vi "Verify Borders.vi"(7 "Column Number":i32, 8 "error in (no error)":errorcluster, 9 "Borders IN":T6={"Title Row Border"={"Line"={"Thickness"=0.5, "Color"=0}, "Column Borders [ ]"=[]}, "Datas Row Borders [ ]"=[]}, 11 "Predefined Borders":T1={"Borders"=0, "Title"={"Thickness"=1.0, "Line"=0, "Background "=16777226}, "Datas"={"Thickness"=0.5, "Line"=0, "Background "=16777215}}) -> (0 "error out":errorcluster, 2 "Borders OUT":T6={"Title Row Border"={"Line"={"Thickness"=0.5, "Color"=0}, "Column Borders [ ]"=[]}, "Datas Row Borders [ ]"=[{"Row"={"#"=0, "to #"=-1}, "Line"={"Thickness"=0.5, "Color"=0}, "Column Borders [ ]"=[]}]}, 4 "ms":u32)   [LabVIEW 2012]
doc: "Version 1.0\nDeveloped by Jean-Marc Simard\nCopyright © 2010, Exaprom Inc.\nAll rights reserved.\nLicense: BSD"
uses:
  Controls/Row Border Title.ctl
  Controls/Cell Border.ctl
  Controls/Row Borders [ ] Datas.ctl
  Controls/Row Predefined borders cluster.ctl
  Controls/Row Predefined borders.ctl
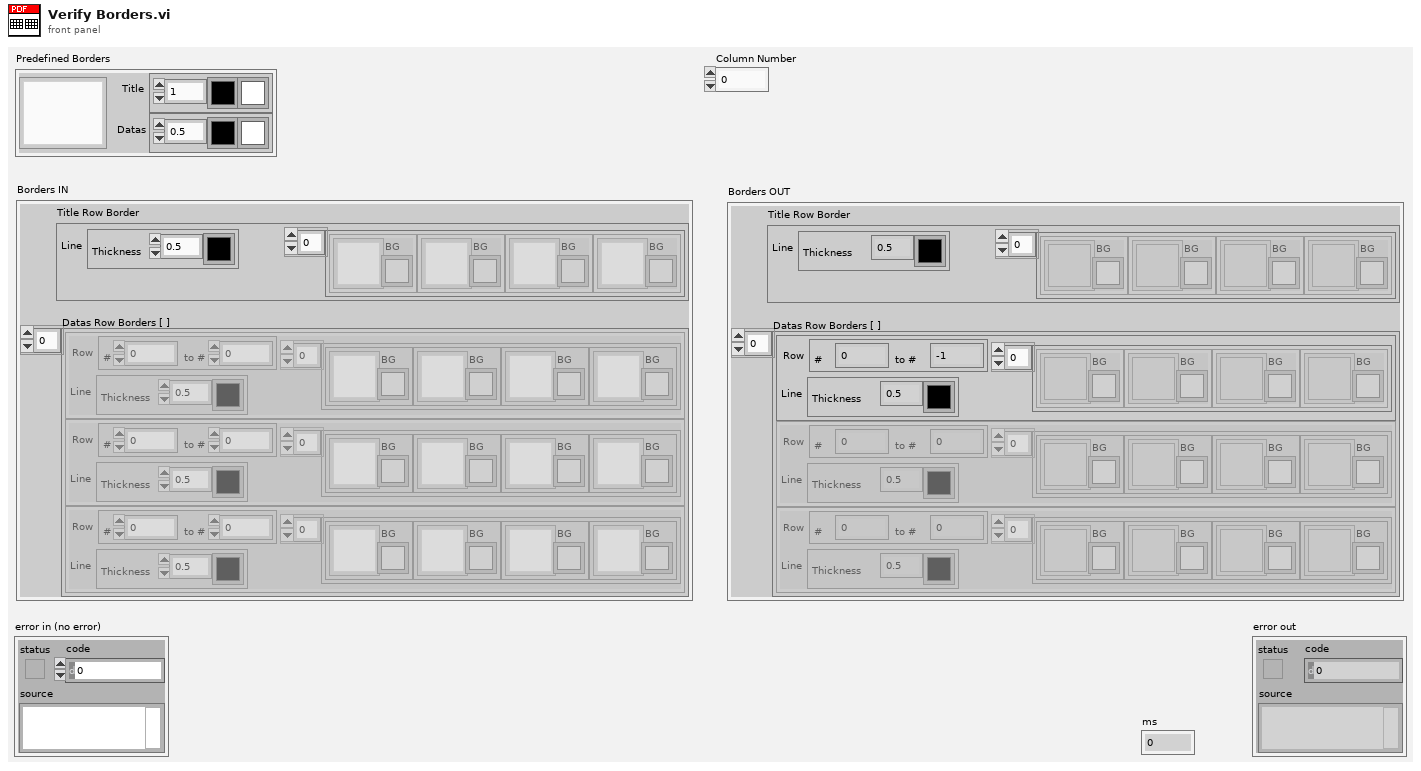
[diagram p1: front panel]
types:
  T1 = typedef "Row Predefined borders cluster.ctl" = cluster{"Borders":T2, "Title":cluster{"Thickness":sgl, "Line":u32, "Background ":u32}, "Datas":cluster{"Thickness":sgl, "Line":u32, "Background ":u32}}
  T2 = typedef "Row Predefined borders.ctl" = u16
  T3 = typedef "Row Border Title.ctl" = cluster{"Line":cluster{"Thickness":sgl, "Color":u32}, "Column Borders [ ]":cluster{"Cell Border":T4, "BG":u32}[]}
  T4 = typedef "Cell Border.ctl" = u16
  T5 = typedef "Row Borders [ ] Datas.ctl" = cluster{"Row":cluster{"#":i16, "to #":i16}, "Line":cluster{"Thickness":sgl, "Color":u32}, "Column Borders [ ]":cluster{"Cell Border":T4, "BG":u32}[]}[]
  T6 = cluster{"Title Row Border":T3, "Datas Row Borders [ ]":T5}
  T7 = cluster{"Row":cluster{"#":i16, "to #":i32}, "Line":cluster{"Thickness":sgl, "Color":u32}, "Column Borders [ ]":cluster{"Cell Border":T4, "BG":u32}[]}
  T8 = cluster{"Row":cluster{"#":i32, "to #":i32}, "Line":cluster{"Thickness":sgl, "Color":u32}, "Column Borders [ ]":cluster{"Cell Border":T4, "BG":u32}[]}
  T9 = cluster{"Row":cluster{"#":i16, "to #":i32}, "Line":cluster{"Thickness":sgl, "Color":u32}, "Column Borders [ ]":cluster{"Cell Border":T4, "BG":u32}[]}[]
  T10 = cluster{"Title Row Border":T3, cluster{"Row":cluster{"#":i16, "to #":i32}, "Line":cluster{"Thickness":sgl, "Color":u32}, "Column Borders [ ]":cluster{"Cell Border":T4, "BG":u32}[]}[]}
  T11 = cluster{"Row":cluster{"#":i32, "to #":i32}, "Line":cluster{"Thickness":sgl, "Color":u32}, "Column Borders [ ]":cluster{"Cell Border":T4, "BG":u32}[]}[]
  T12 = cluster{"Title Row Border":T3, cluster{"Row":cluster{"#":i32, "to #":i32}, "Line":cluster{"Thickness":sgl, "Color":u32}, "Column Borders [ ]":cluster{"Cell Border":T4, "BG":u32}[]}[]}
  T13 = cluster{"Row":cluster{"#":i16, "to #":i16}, "Line":cluster{"Thickness":sgl, "Color":u32}, "Column Borders [ ]":cluster{"Cell Border":T4, "BG":u32}[]}
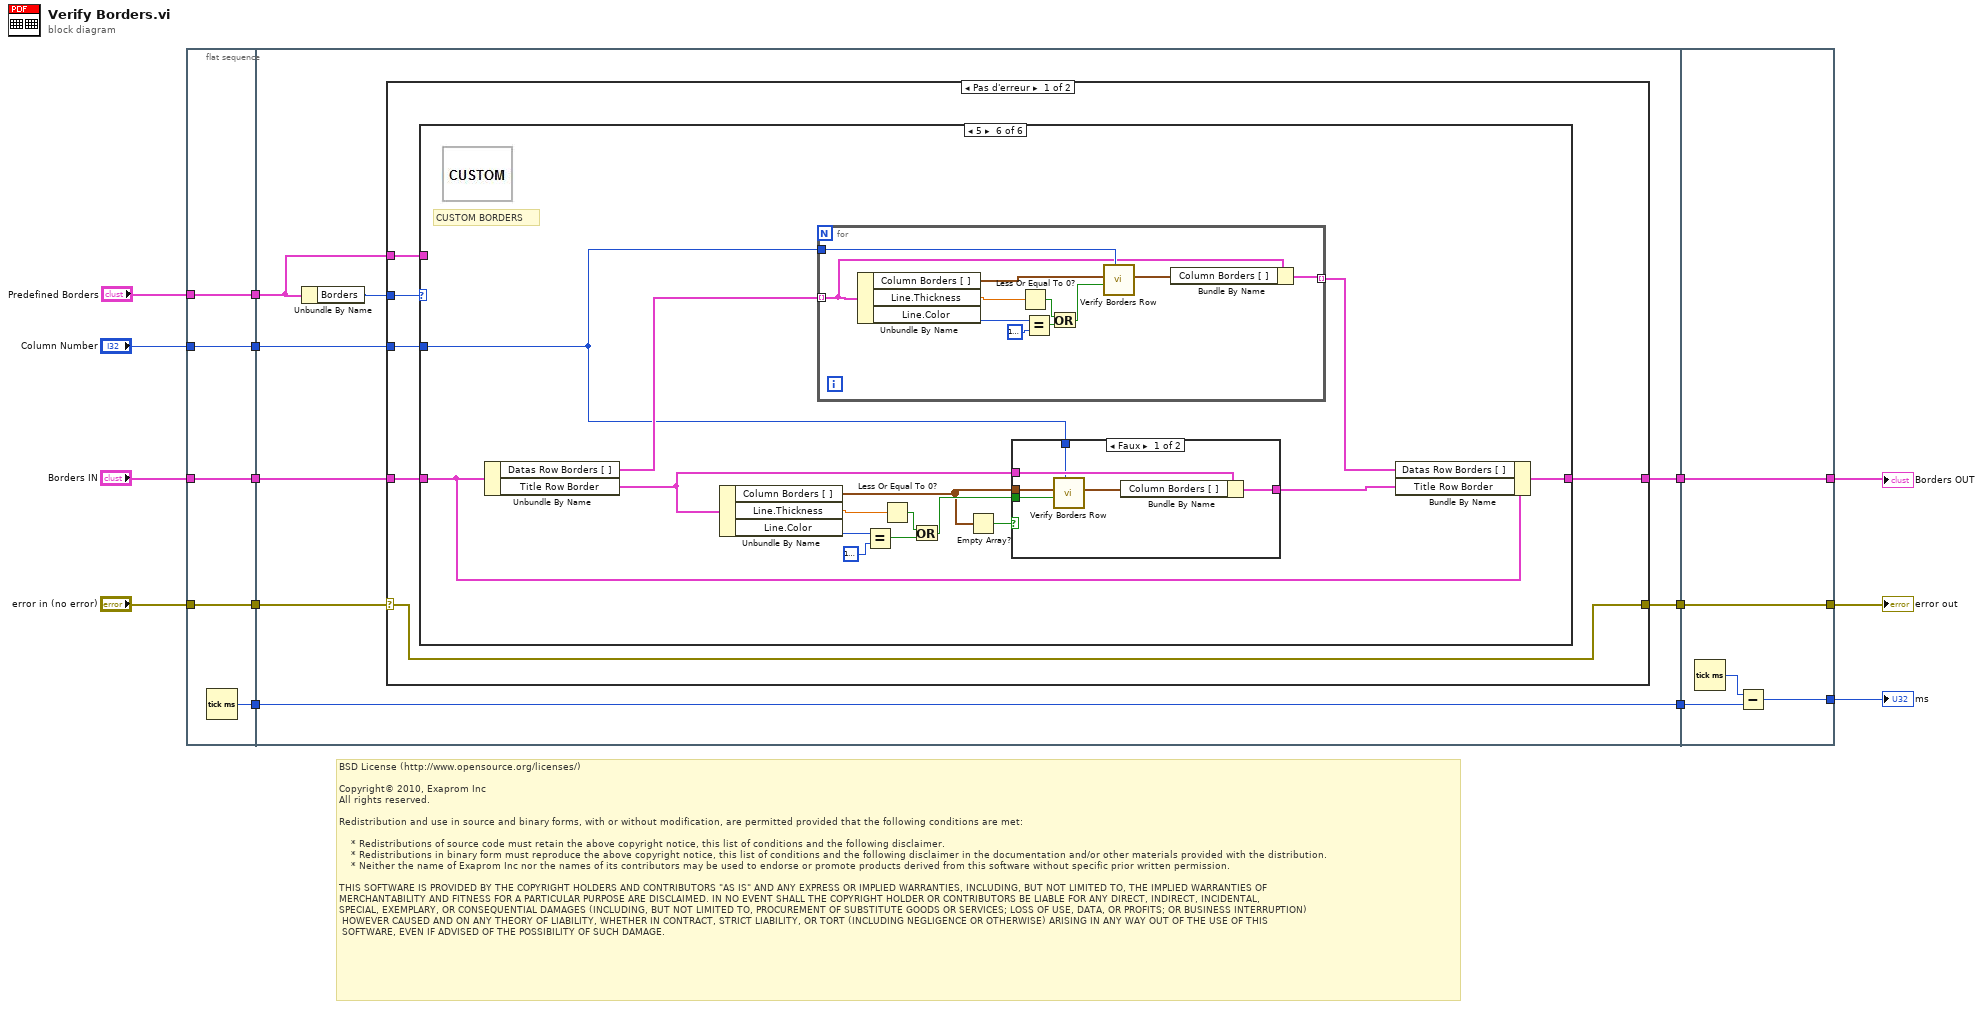
[diagram p0: block diagram]
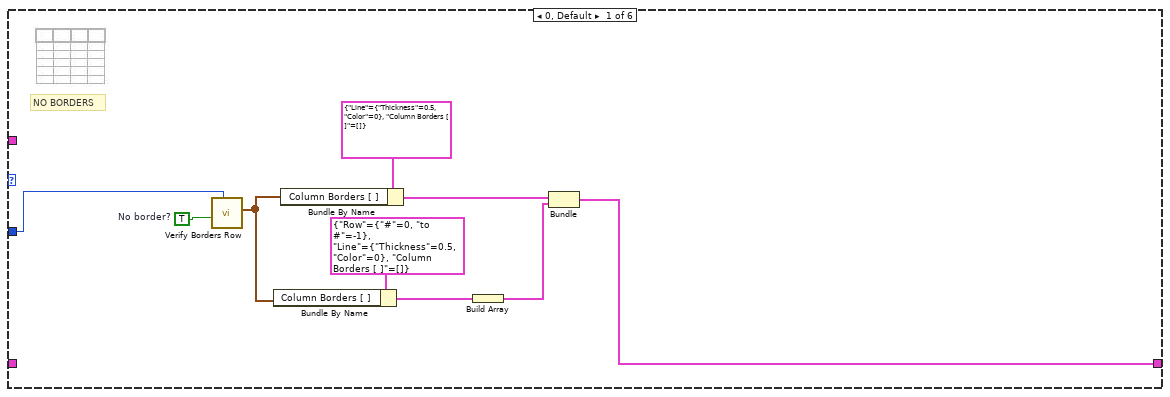
[diagram p2: hidden frame]
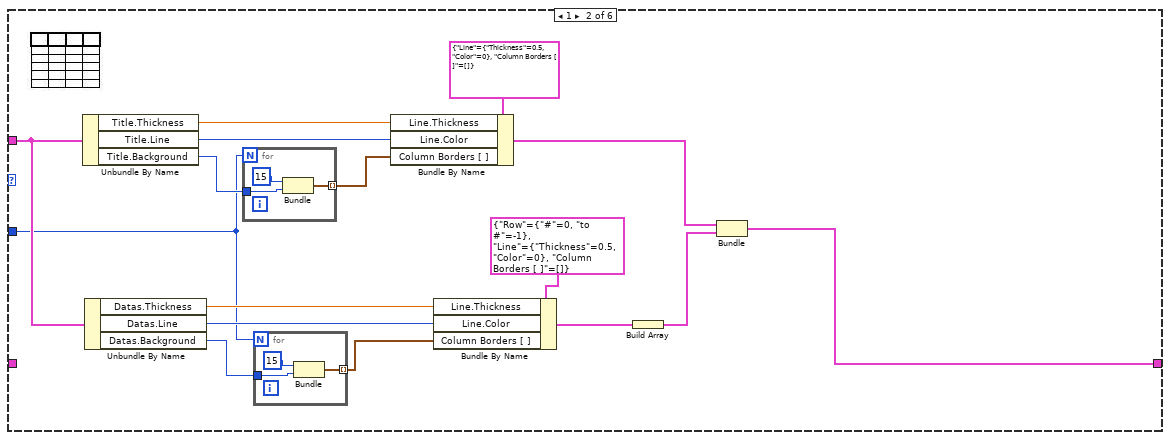
[diagram p3: hidden frame]
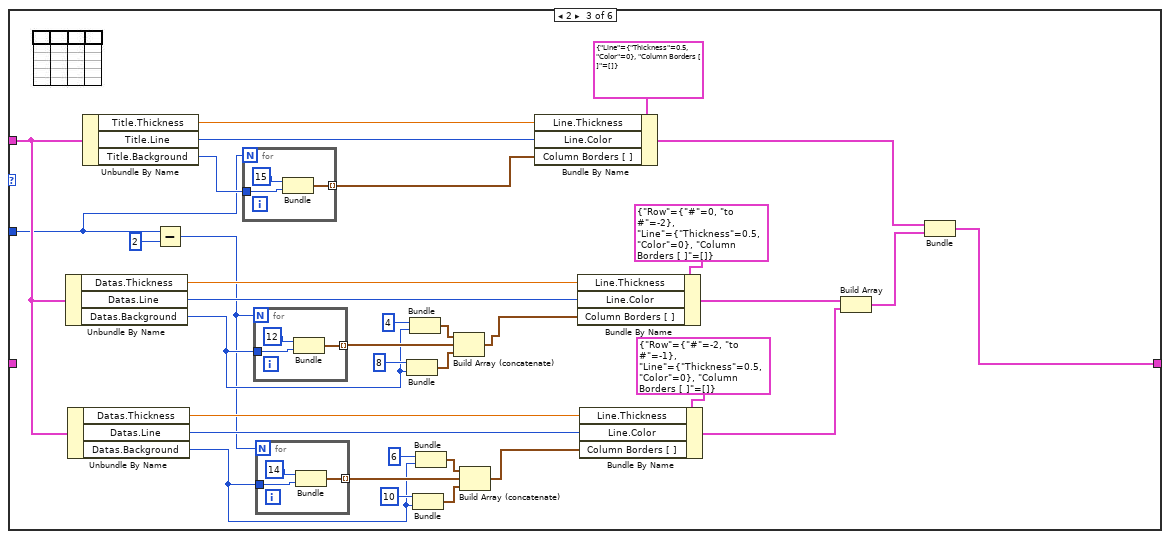
[diagram p4: hidden frame]
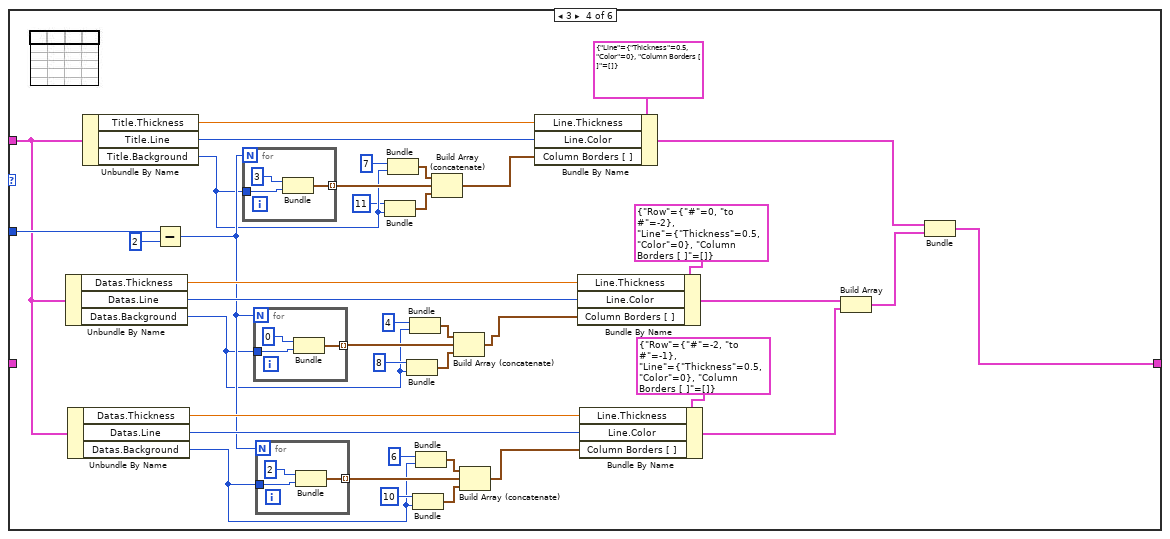
[diagram p5: hidden frame]
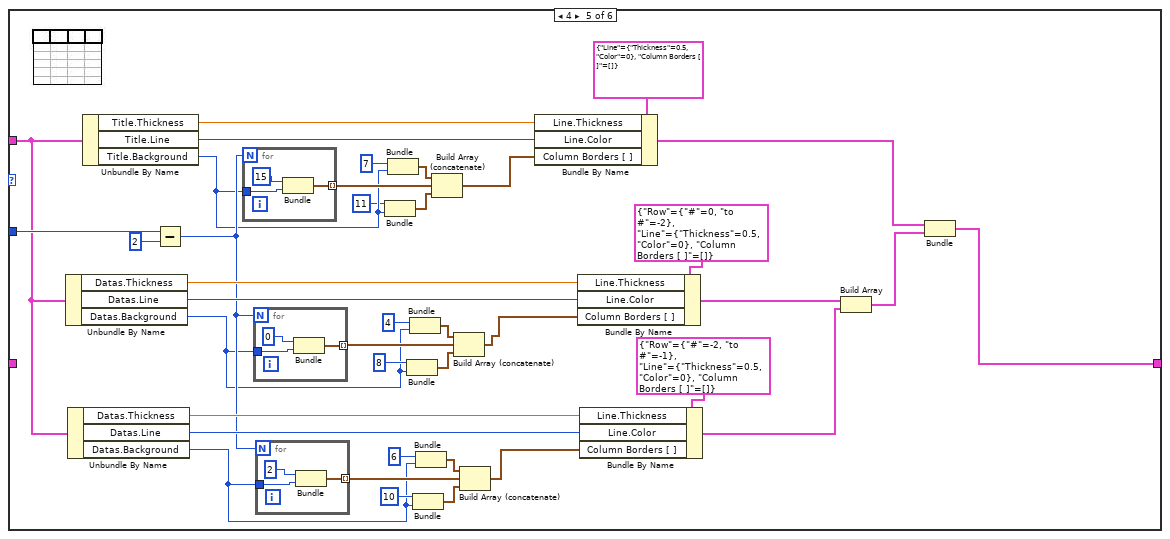
[diagram p6: hidden frame]
diagram:
  # "BSD License (http://www.opensource.org/licenses/)\n\nCopyright© 2010, Exaprom Inc\nAll rights reserved.\n\nRedistribution and use in source and binary forms, with or without modification, are permitted provided that the following conditions are met:\n\n    * Redistributions of source code must retain the above copyright notice, this list of conditions and the following disclaimer.\n    * Redistributions in binary form must reproduce the above copyright notice, this list of conditions and the following disclaimer in the documentation and/or other materials provided with the distribution.\n    * Neither the name of Exaprom Inc nor the names of its contributors may be used to endorse or promote products derived from this software without specific prior written permission.\n\nTHIS SOFTWARE IS PROVIDED BY THE COPYRIGHT HOLDERS AND CONTRIBUTORS \"AS IS\" AND ANY EXPRESS OR IMPLIED WARRANTIES, INCLUDING, BUT NOT LIMITED TO, THE IMPLIED WARRANTIES OF \nMERCHANTABILITY AND FITNESS FOR A PARTICULAR PURPOSE ARE DISCLAIMED. IN NO EVENT SHALL THE COPYRIGHT HOLDER OR CONTRIBUTORS BE LIABLE FOR ANY DIRECT, INDIRECT, INCIDENTAL,\nSPECIAL, EXEMPLARY, OR CONSEQUENTIAL DAMAGES (INCLUDING, BUT NOT LIMITED TO, PROCUREMENT OF SUBSTITUTE GOODS OR SERVICES; LOSS OF USE, DATA, OR PROFITS; OR BUSINESS INTERRUPTION)\n HOWEVER CAUSED AND ON ANY THEORY OF LIABILITY, WHETHER IN CONTRACT, STRICT LIABILITY, OR TORT (INCLUDING NEGLIGENCE OR OTHERWISE) ARISING IN ANY WAY OUT OF THE USE OF THIS\n SOFTWARE, EVEN IF ADVISED OF THE POSSIBILITY OF SUCH DAMAGE."
  n1 = flat-sequence {
    tunnel: "Predefined Borders" -> [w17]
    tunnel: "Borders IN" -> [w18]
    tunnel: "Column Number" -> [w19]
    tunnel: "error in (no error)" -> [w20]
    tunnel: [w20] -> w9
    tunnel: [w19] -> w8
    tunnel: [w18] -> w7
    tunnel: [w17] -> w6
    tunnel: [w16] -> w2
    tunnel: w9 -> [w28]
    tunnel: w8 -> [w26]
    tunnel: w7 -> [w25]
    tunnel: w6 -> [w22]
    tunnel: [w27] -> w5
    tunnel: [w24] -> w4
    tunnel: [w21] -> w3
    tunnel: w2 -> [w21]
    tunnel: [w243] -> w11
    tunnel: [w244] -> w14
    tunnel: w5 -> [w244]
    tunnel: w4 -> [w243]
    tunnel: w3 -> [w241]
    tunnel: [w240] -> w1
    frame #0 {
      n2 = Tick Count (ms)() -> (millisecond timer value=w16:u32)
    }
    frame #1 {
      n3 = Unbundle By Name(w22) -> ("Borders"=w23:T2)
      n4 = case shown="Pas d'erreur" w28 {
        selector: w28 -> [w29 w239]
        tunnel: [w29 w239] -> w27
        tunnel: w26 -> [w32 _]
        tunnel: [w33 w238] -> w24
        tunnel: w25 -> [w34 w238]
        tunnel: w23 -> [w31 _]
        tunnel: w22 -> [w30 _]
        frame No Error {
          n5 = case shown="5" w31 {
            tunnel: w34 -> [_ _ _ _ _ w212]
            tunnel: [w37 w55 w95 w143 w191 w209] -> w33
            tunnel: w32 -> [w35 w44 w67 w133 w181 w208]
            tunnel: w30 -> [_ w49 w86 w132 w180 _]
            frame 0, Default {
              w43 = TRUE  # No border?
              # "NO BORDERS"
              n6 = call "Verify Borders Row.vi"("Column Number"=w35, "No border?"=w43) -> ("Column Borders OUT [ ]"=w41:cluster{"Cell Border":T4, "BG":u32}[])  [unwired: 2 in, 7 out]
              n7 = Bundle By Name(cluster=T7 {"Row"={"#"=0, "to #"=-1}, "Line"={"Thickness"=0.5, "Color"=0}, "Column Borders [ ]"=[]} ("Row Borders"), "Column Borders [ ]"=w41) -> (w38:T7)
              n8 = Bundle By Name(cluster=T3 {"Line"={"Thickness"=0.5, "Color"=0}, "Column Borders [ ]"=[]} ("Title Row Border"), "Column Borders [ ]"=w41) -> (w39:T3)
              n9 = Build Array(w38) -> (w36:T9)
              n10 = Bundle("Title Row Border"=w39, w36) -> (w37:T10)  [unwired: 1 out]
            }
            frame 1 {
              n11 = Unbundle By Name(w49) -> ("Title.Thickness"=w53:sgl, "Title.Line"=w52:u32, "Title.Background"=w51:u32)
              n12 = Unbundle By Name(w49) -> ("Datas.Thickness"=w48:sgl, "Datas.Line"=w47:u32, "Datas.Background"=w46:u32)
              n13 = for {
                N: w44 -> [_]
                tunnel: w51 -> [w64]
                tunnel: [w63] -> w50 mode=indexing
                n14 = Bundle(15, "Background"=w64) -> (w63:cluster{i32, "Background ":u32})  [unwired: 1 out]
              }
              n15 = for {
                N: w44 -> [_]
                tunnel: w46 -> [w61]
                tunnel: [w60] -> w45 mode=indexing
                n16 = Bundle(15, "Background"=w61) -> (w60:cluster{i32, "Background ":u32})  [unwired: 1 out]
              }
              n17 = Bundle By Name(cluster=T3 {"Line"={"Thickness"=0.5, "Color"=0}, "Column Borders [ ]"=[]} ("Title Row Border"), "Line.Thickness"=w53, "Line.Color"=w52, "Column Borders [ ]"=w50) -> (w57:T3)
              n18 = Bundle By Name(cluster=T7 {"Row"={"#"=0, "to #"=-1}, "Line"={"Thickness"=0.5, "Color"=0}, "Column Borders [ ]"=[]} ("Row Borders"), "Line.Thickness"=w48, "Line.Color"=w47, "Column Borders [ ]"=w45) -> (w56:T7)
              n19 = Build Array(w56) -> (w54:T9)
              n20 = Bundle("Title Row Border"=w57, w54) -> (w55:T10)  [unwired: 1 out]
            }
            frame 2 {
              n21 = Unbundle By Name(w86) -> ("Datas.Thickness"=w91:sgl, "Datas.Line"=w90:u32, "Datas.Background"=w76:u32)
              n22 = Unbundle By Name(w86) -> ("Datas.Thickness"=w88:sgl, "Datas.Line"=w89:u32, "Datas.Background"=w69:u32)
              n23 = Unbundle By Name(w86) -> ("Title.Thickness"=w93:sgl, "Title.Line"=w92:u32, "Title.Background"=w83:u32)
              n24 = Subtract(x=w67, y=2) -> (x-y=w66:i32)
              n25 = for {
                N: w67 -> [_]
                tunnel: w83 -> [w107]
                tunnel: [w106] -> w68 mode=indexing
                n26 = Bundle(15, "Background"=w107) -> (w106:cluster{i32, "Background ":u32})  [unwired: 1 out]
              }
              n27 = for {
                N: w66 -> [_]
                tunnel: w76 -> [w104]
                tunnel: [w103] -> w78 mode=indexing
                n28 = Bundle(12, "Background"=w104) -> (w103:cluster{i32, "Background ":u32})  [unwired: 1 out]
              }
              n29 = for {
                N: w66 -> [_]
                tunnel: w69 -> [w101]
                tunnel: [w100] -> w71 mode=indexing
                n30 = Bundle(14, "Background"=w101) -> (w100:cluster{i32, "Background ":u32})  [unwired: 1 out]
              }
              n31 = Bundle(8, "Background"=w76) -> (w80:cluster{i32, "Background ":u32})  [unwired: 1 out]
              n32 = Bundle(4, "Background"=w76) -> (w79:cluster{i32, "Background ":u32})  [unwired: 1 out]
              n33 = Bundle(10, "Background"=w69) -> (w74:cluster{i32, "Background ":u32})  [unwired: 1 out]
              n34 = Bundle(6, "Background"=w69) -> (w75:cluster{i32, "Background ":u32})  [unwired: 1 out]
              n35 = Build Array (concatenate)(w79, w78, w80) -> (w77:cluster{i32, "Background ":u32}[])
              n36 = Build Array (concatenate)(w75, w71, w74) -> (w70:cluster{i32, "Background ":u32}[])
              n37 = Bundle By Name(cluster=T3 {"Line"={"Thickness"=0.5, "Color"=0}, "Column Borders [ ]"=[]} ("Title Row Border"), "Line.Thickness"=w93, "Line.Color"=w92, "Column Borders [ ]"=w68) -> (w97:T3)
              n38 = Bundle By Name(cluster=T7 {"Row"={"#"=0, "to #"=-2}, "Line"={"Thickness"=0.5, "Color"=0}, "Column Borders [ ]"=[]} ("Row Borders"), "Line.Thickness"=w91, "Line.Color"=w90, "Column Borders [ ]"=w77) -> (w96:T7)
              n39 = Bundle By Name(cluster=T8 {"Row"={"#"=-2, "to #"=-1}, "Line"={"Thickness"=0.5, "Color"=0}, "Column Borders [ ]"=[]} ("Row Borders"), "Line.Thickness"=w88, "Line.Color"=w89, "Column Borders [ ]"=w70) -> (w85:T8)
              n40 = Build Array(w96, w85) -> (w94:T11)
              n41 = Bundle("Title Row Border"=w97, w94) -> (w95:T12)  [unwired: 1 out]
            }
            frame 3 {
              n42 = Unbundle By Name(w132) -> ("Datas.Thickness"=w138:sgl, "Datas.Line"=w137:u32, "Datas.Background"=w116:u32)
              n43 = Unbundle By Name(w132) -> ("Datas.Thickness"=w135:sgl, "Datas.Line"=w136:u32, "Datas.Background"=w109:u32)
              n44 = Unbundle By Name(w132) -> ("Title.Thickness"=w141:sgl, "Title.Line"=w140:u32, "Title.Background"=w127:u32)
              n45 = Subtract(x=w133, y=2) -> (x-y=w130:i32)
              n46 = for {
                N: w130 -> [_]
                tunnel: w127 -> [w155]
                tunnel: [w154] -> w139 mode=indexing
                n47 = Bundle(3, "Background"=w155) -> (w154:cluster{i32, "Background ":u32})  [unwired: 1 out]
              }
              n48 = for {
                N: w130 -> [_]
                tunnel: w116 -> [w152]
                tunnel: [w151] -> w118 mode=indexing
                n49 = Bundle(0, "Background"=w152) -> (w151:cluster{i32, "Background ":u32})  [unwired: 1 out]
              }
              n50 = for {
                N: w130 -> [_]
                tunnel: w109 -> [w149]
                tunnel: [w148] -> w111 mode=indexing
                n51 = Bundle(2, "Background"=w149) -> (w148:cluster{i32, "Background ":u32})  [unwired: 1 out]
              }
              n52 = Bundle(11, "Background"=w127) -> (w125:cluster{i32, "Background ":u32})  [unwired: 1 out]
              n53 = Bundle(7, "Background"=w127) -> (w126:cluster{i32, "Background ":u32})  [unwired: 1 out]
              n54 = Bundle(8, "Background"=w116) -> (w120:cluster{i32, "Background ":u32})  [unwired: 1 out]
              n55 = Bundle(4, "Background"=w116) -> (w119:cluster{i32, "Background ":u32})  [unwired: 1 out]
              n56 = Bundle(10, "Background"=w109) -> (w114:cluster{i32, "Background ":u32})  [unwired: 1 out]
              n57 = Bundle(6, "Background"=w109) -> (w115:cluster{i32, "Background ":u32})  [unwired: 1 out]
              n58 = Build Array (concatenate)(w126, w139, w125) -> (w128:cluster{i32, "Background ":u32}[])
              n59 = Build Array (concatenate)(w119, w118, w120) -> (w117:cluster{i32, "Background ":u32}[])
              n60 = Build Array (concatenate)(w115, w111, w114) -> (w110:cluster{i32, "Background ":u32}[])
              n61 = Bundle By Name(cluster=T3 {"Line"={"Thickness"=0.5, "Color"=0}, "Column Borders [ ]"=[]} ("Title Row Border"), "Line.Thickness"=w141, "Line.Color"=w140, "Column Borders [ ]"=w128) -> (w145:T3)
              n62 = Bundle By Name(cluster=T7 {"Row"={"#"=0, "to #"=-2}, "Line"={"Thickness"=0.5, "Color"=0}, "Column Borders [ ]"=[]} ("Row Borders"), "Line.Thickness"=w138, "Line.Color"=w137, "Column Borders [ ]"=w117) -> (w144:T7)
              n63 = Bundle By Name(cluster=T8 {"Row"={"#"=-2, "to #"=-1}, "Line"={"Thickness"=0.5, "Color"=0}, "Column Borders [ ]"=[]} ("Row Borders"), "Line.Thickness"=w135, "Line.Color"=w136, "Column Borders [ ]"=w110) -> (w131:T8)
              n64 = Build Array(w144, w131) -> (w142:T11)
              n65 = Bundle("Title Row Border"=w145, w142) -> (w143:T12)  [unwired: 1 out]
            }
            frame 4 {
              n66 = Unbundle By Name(w180) -> ("Datas.Thickness"=w186:sgl, "Datas.Line"=w185:u32, "Datas.Background"=w164:u32)
              n67 = Unbundle By Name(w180) -> ("Datas.Thickness"=w183:sgl, "Datas.Line"=w184:u32, "Datas.Background"=w157:u32)
              n68 = Unbundle By Name(w180) -> ("Title.Thickness"=w189:sgl, "Title.Line"=w188:u32, "Title.Background"=w175:u32)
              n69 = Subtract(x=w181, y=2) -> (x-y=w178:i32)
              n70 = for {
                N: w178 -> [_]
                tunnel: w175 -> [w203]
                tunnel: [w202] -> w187 mode=indexing
                n71 = Bundle(15, "Background"=w203) -> (w202:cluster{i32, "Background ":u32})  [unwired: 1 out]
              }
              n72 = for {
                N: w178 -> [_]
                tunnel: w164 -> [w200]
                tunnel: [w199] -> w166 mode=indexing
                n73 = Bundle(0, "Background"=w200) -> (w199:cluster{i32, "Background ":u32})  [unwired: 1 out]
              }
              n74 = for {
                N: w178 -> [_]
                tunnel: w157 -> [w197]
                tunnel: [w196] -> w159 mode=indexing
                n75 = Bundle(2, "Background"=w197) -> (w196:cluster{i32, "Background ":u32})  [unwired: 1 out]
              }
              n76 = Bundle(11, "Background"=w175) -> (w173:cluster{i32, "Background ":u32})  [unwired: 1 out]
              n77 = Bundle(7, "Background"=w175) -> (w174:cluster{i32, "Background ":u32})  [unwired: 1 out]
              n78 = Bundle(8, "Background"=w164) -> (w168:cluster{i32, "Background ":u32})  [unwired: 1 out]
              n79 = Bundle(4, "Background"=w164) -> (w167:cluster{i32, "Background ":u32})  [unwired: 1 out]
              n80 = Bundle(10, "Background"=w157) -> (w162:cluster{i32, "Background ":u32})  [unwired: 1 out]
              n81 = Bundle(6, "Background"=w157) -> (w163:cluster{i32, "Background ":u32})  [unwired: 1 out]
              n82 = Build Array (concatenate)(w174, w187, w173) -> (w176:cluster{i32, "Background ":u32}[])
              n83 = Build Array (concatenate)(w167, w166, w168) -> (w165:cluster{i32, "Background ":u32}[])
              n84 = Build Array (concatenate)(w163, w159, w162) -> (w158:cluster{i32, "Background ":u32}[])
              n85 = Bundle By Name(cluster=T3 {"Line"={"Thickness"=0.5, "Color"=0}, "Column Borders [ ]"=[]} ("Title Row Border"), "Line.Thickness"=w189, "Line.Color"=w188, "Column Borders [ ]"=w176) -> (w193:T3)
              n86 = Bundle By Name(cluster=T7 {"Row"={"#"=0, "to #"=-2}, "Line"={"Thickness"=0.5, "Color"=0}, "Column Borders [ ]"=[]} ("Row Borders"), "Line.Thickness"=w186, "Line.Color"=w185, "Column Borders [ ]"=w165) -> (w192:T7)
              n87 = Bundle By Name(cluster=T8 {"Row"={"#"=-2, "to #"=-1}, "Line"={"Thickness"=0.5, "Color"=0}, "Column Borders [ ]"=[]} ("Row Borders"), "Line.Thickness"=w183, "Line.Color"=w184, "Column Borders [ ]"=w158) -> (w179:T8)
              n88 = Build Array(w192, w179) -> (w190:T11)
              n89 = Bundle("Title Row Border"=w193, w190) -> (w191:T12)  [unwired: 1 out]
            }
            frame 5 {
              # "CUSTOM BORDERS"
              n90 = Unbundle By Name(w212) -> ("Datas Row Borders [ ]"=w219:T5, "Title Row Border"=w213:T3)
              n91 = Unbundle By Name(w213) -> ("Column Borders [ ]"=w206:cluster{"Cell Border":T4, "BG":u32}[], "Line.Thickness"=w215:sgl, "Line.Color"=w214:u32)
              n92 = for {
                tunnel: w219 -> [w227] mode=indexing
                tunnel: [w229] -> w211 mode=indexing
                tunnel: w208 -> [w228]
                n93 = Unbundle By Name(w227) -> ("Column Borders [ ]"=w233:cluster{"Cell Border":T4, "BG":u32}[], "Line.Thickness"=w235:sgl, "Line.Color"=w236:u32)
                n94 = Less Or Equal To 0?(x=w235) -> (x <= 0?=w230:bool)
                n95 = Equal?(x=w236, y=u32 16777225 ("Color Box")) -> (x = y?=w234:bool)
                n96 = Or(x=w230, y=w234) -> (x .or. y?=w232:bool)
                n97 = call "Verify Borders Row.vi"("Column Number"=w228, "No border?"=w232, "Column Borders IN [ ]"=w233) -> ("Column Borders OUT [ ]"=w231:cluster{"Cell Border":T4, "BG":u32}[])  [unwired: 1 in, 7 out]
                n98 = Bundle By Name(cluster=w227, "Column Borders [ ]"=w231) -> (w229:T13)
              }
              n99 = Equal?(x=w214, y=u32 16777225 ("Color Box")) -> (x = y?=w216:bool)
              n100 = Less Or Equal To 0?(x=w215) -> (x <= 0?=w218:bool)
              n101 = Or(x=w218, y=w216) -> (x .or. y?=w217:bool)
              n102 = Empty Array?(array=w206) -> (empty?=w205:bool)
              n103 = case shown="Faux" w205 {
                tunnel: w217 -> [w224 _]
                tunnel: w213 -> [w223 w226]
                tunnel: [w222 w226] -> w210
                tunnel: w208 -> [w221 _]
                tunnel: w206 -> [w220 _]
                frame False {
                  n104 = call "Verify Borders Row.vi"("Column Number"=w221, "No border?"=w224, "Column Borders IN [ ]"=w220) -> ("Column Borders OUT [ ]"=w225:cluster{"Cell Border":T4, "BG":u32}[])  [unwired: 1 in, 7 out]
                  n105 = Bundle By Name(cluster=w223, "Column Borders [ ]"=w225) -> (w222:T3)
                }
                frame True {
                }
              }
              n106 = Bundle By Name(cluster=w212, "Datas Row Borders [ ]"=w211, "Title Row Border"=w210) -> (w209:T6)
            }
          }
        }
        frame Error {
        }
      }
    }
    frame #2 {
      n107 = Tick Count (ms)() -> (millisecond timer value=w242:u32)
      n108 = Subtract(x=w242, y=w241) -> (x-y=w240:u32)
    }
  }
  "error out" <- w14
  "Borders OUT" <- w11
  "ms" <- w1
